vi "Generate Extension Values.vi"(3 "Height":u32) -> (0 "Heights":dbl[](array[numeric]), 1 "Origins":cluster{i32, dbl}[](array[cluster]))   [LabVIEW 2013]
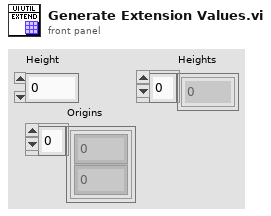
[diagram p1: front panel]
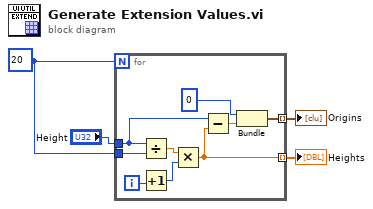
[diagram p0: block diagram]
diagram:
  w4 = 20
  n1 = for {
    N: w4 -> [_]
    tunnel: w4 -> [w9]
    tunnel: "Height" -> [w8]
    tunnel: [w6] -> w2 mode=indexing
    tunnel: [w5] -> w1 mode=indexing
    i -> [w7]
    n2 = Divide(x=w8, y=w9) -> (x/y=w13:dbl)
    n3 = Increment(x=w7) -> (x+1=w10:i32)
    n4 = Multiply(x=w13, y=w10) -> (x*y=w5:dbl)
    n5 = Subtract(x=w8, y=w5) -> (x-y=w11:dbl)
    n6 = Bundle(0, w11) -> (w6:cluster{i32, dbl})  [unwired: 1 in]
  }
  "Origins" <- w2
  "Heights" <- w1
